vi "InitPreconfiguredSleeveData.vi"   [LabVIEW 2013]
uses:
  GlobalVariables/PreconfiguredSleeveData.vi
types:
  T1 = cluster{"sleeveLength":string, "sleeveDiameter":string, "sleeveThickness":string}
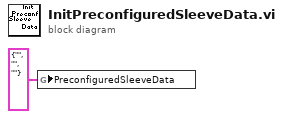
[diagram p0: block diagram]
diagram:
  n1 = global write "PreconfiguredSleeveData.vi" "PreconfiguredSleeveData"(T1 {"sleeveLength"="", "sleeveDiameter"="", "sleeveThickness"=""} ("PreconfiguredSleeveData")) -> ()
